vi "Submit Order.vi"(8 "error in (no error)":errorcluster, 10 "Order.lvclass":refnum<class "Order.lvclass">, 11 "Customer in":refnum<class "Customer.lvclass">) -> (0 "error out":errorcluster, 3 "Customer out":refnum<class "Customer.lvclass">)   [LabVIEW 2023, in "Customer.lvlib" / "Customer.lvclass"]
doc: "Method VI for customer to submit a particular order."
uses:
  Customer.lvclass
  c:/dev/_r/4/eng/lv-core/lvpostprocessingd/lv_mc_x86_64/dist_i386/vi.lib/ActorFramework/Actor/Actor.lvclass
  Order/Order.lvclass
  <vilib>/ActorFramework/Actor/Actor.lvclass/Actor.ctl
  <vilib>/ActorFramework/Message Enqueuer/Message Enqueuer.lvclass/Message Enqueuer.ctl
  Person Messages/Show or Hide Front Panel Msg/Show or Hide Front Panel Msg.lvclass/Show or Hide Front Panel Msg.ctl
  Work Dispatcher Messages/Add Task Msg/Add Task Msg.lvclass/Add Task Msg.ctl
  <vilib>/ActorFramework/Message Enqueuer/Init from Existing Queue.vi
  <vilib>/ActorFramework/Message Enqueuer/Enqueue.vi
  Person Messages/Show or Hide Front Panel Msg/Show or Hide Front Panel Msg.lvclass
  c:/dev/_r/4/eng/lv-core/lvpostprocessingd/lv_mc_x86_64/dist_i386/vi.lib/ActorFramework/Message/Message.lvclass
  Work Dispatcher Messages/Add Task Msg/Add Task Msg.lvclass
  <vilib>/ActorFramework/Message Priority Queue/Priority Enqueue.vi
  <vilib>/ActorFramework/Message Enqueuer/Message Enqueuer.lvclass
  <vilib>/ActorFramework/Actor/Actor.lvclass
panel:
  in  "Ordered":string="Ordered"
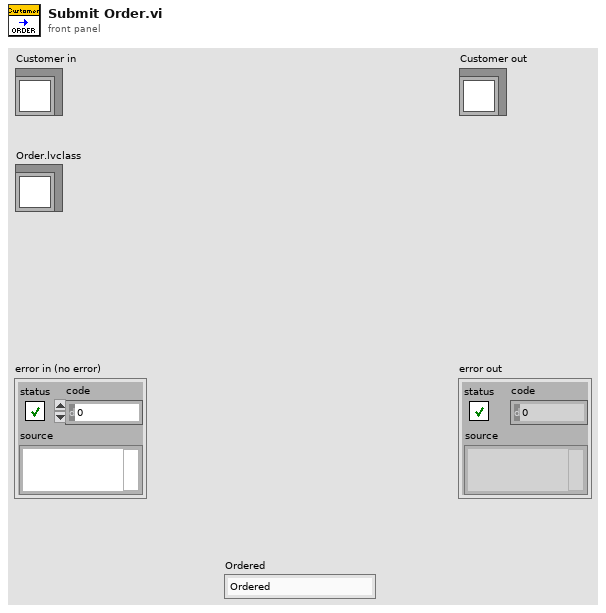
[diagram p1: front panel]
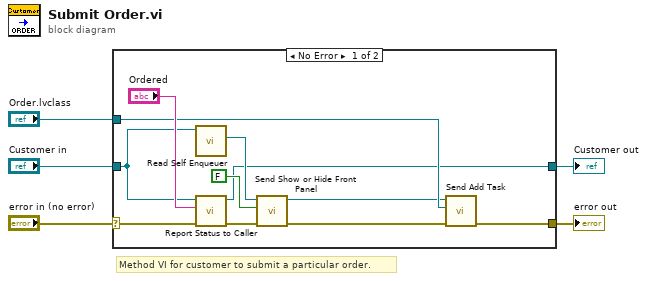
[diagram p0: block diagram]
diagram:
  # "Method VI for customer to submit a particular order."
  n1 = case shown="No Error" "error in (no error)" {
    selector: "error in (no error)" -> [w6 w18]
    tunnel: [w8 w18] -> w4
    tunnel: [w7 w17] -> w2
    tunnel: "Customer in" -> [w15 w17]
    tunnel: "Order.lvclass" -> [w14 _]
    frame No Error {
      n2 = call <vilib>:"Read Self Enqueuer.vi"("Actor"=w15) -> ("Self Enqueuer"=w12:refnum<class "Message Enqueuer.lvclass">)  [unwired: 10 in]
      n3 = call-dynamic "Report Status to Caller.vi"("error in"=w6, "Status"="Ordered", "Customer in"=w15) -> ("error out"=w10:errorcluster, "Customer out"=w7:refnum<class "Customer.lvclass">)  [unwired: 7 in]
      n4 = call "Send Show or Hide Front Panel.vi"("error in (no error)"=w10, "Show Front Panel?"=FALSE, "Message Enqueuer"=w12) -> ("error out"=w9:errorcluster, "Message Enqueuer out"=w11:refnum<class "Message Enqueuer.lvclass">)  [unwired: 7 in]
      n5 = call "Send Add Task.vi"("error in (no error)"=w9, "Task"=w14, "Message Enqueuer"=w11) -> ("error out"=w8:errorcluster)  [unwired: 7 in, 1 out]
    }
    frame Error {
    }
  }
  "error out" <- w4
  "Customer out" <- w2
